vi "Configure VIs.Blacklist.vi"(8 "error in (no error)":errorcluster, 10 "Blacklist VIs":string[](array[string])=["Configure VIs for Development.vi", "Configure VIs for Execution.vi"], 11 "VI reference in":refnum<vi>) -> (0 "error out":errorcluster, 2 "valid?":bool, 3 "VI reference out":refnum<vi>)   [LabVIEW 2017]
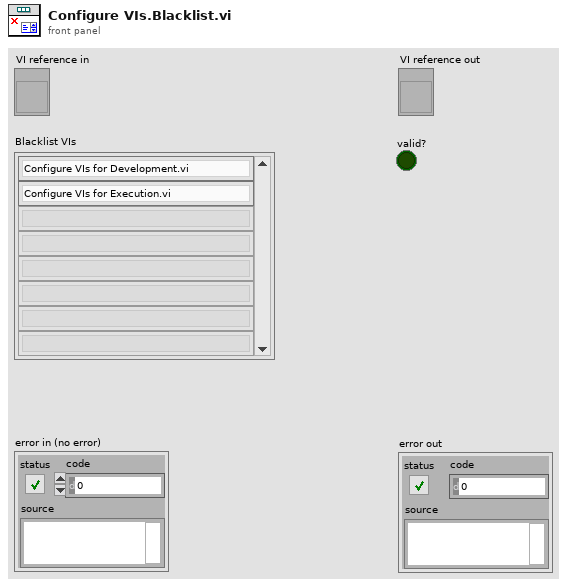
[diagram p1: front panel]
types:
  T1 = enum32{"invalid VI type", "Standard VI", "Control VI", "Global VI", "Polymorphic VI", "Configuration VI", "SubSystem", "Facade VI", "Method VI", "Statechart Diagram VI"}
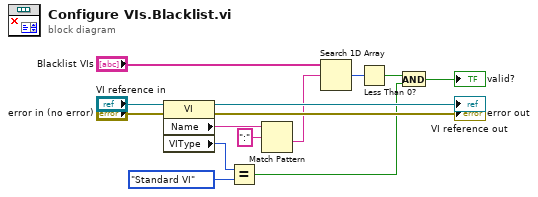
[diagram p0: block diagram]
diagram:
  n1 = property class="VI"(reference="VI reference in", error in="error in (no error)") -> (reference out=→"VI reference out":refnum<vi>, error out=→"error out":errorcluster, "Name"=w2:string, "VIType"=w11:T1)
  n2 = Equal?(x=w11, y=T1."Standard VI" ("VI Type")) -> (x = y?=w4:bool)
  n3 = Match Pattern(string=w2, regular expression=":") -> (after substring=w1:string)  [unwired: 1 in, 3 out]
  n4 = Search 1D Array(1D array="Blacklist VIs", element=w1) -> (index of element=w9:i32)  [unwired: 1 in]
  n5 = Less Than 0?(x=w9) -> (x < 0?=w8:bool)
  n6 = And(x=w8, y=w4) -> (x .and. y?=→"valid?":bool)
